vi "Parse Wiki.vi"(8 "error in":errorcluster, 9 "Parse from":enum16{"Proposal HTML:", "Proposal cluster"}(ring), 10 "Proposal Data":T2, 11 "Proposal document":path=path "C:/Users/l121767/Dropbox/Projects/FAIR/Project files/Proposal/National High Magnetic Field Laboratory - Users Program.html") -> (0 "error out":errorcluster, 3 "Puject  JSON":string)   [LabVIEW 2020]
uses:
  Utilities/iCalendar/Extract iCalendar String.ctl
  55103850-15ef-4a18-9388-7b0eadcdd449.vi
  <vilib>/JDP Science/JSONtext/Variant to JSON Text.vi
  <vilib>/JDP Science/JSONtext/LVClass Serializer/JSONtext LVClass Serializer.lvclass
panel:
  in  "OSF sub-project":T1={"data"={"type"="nodes", "attributes"={"title"="", "description"="", "public"=FALSE, "category"=""}}}
  in  "OSF Wiki":T3={"data"={"type"="wikis", "attributes"={"name"="", "content"=""}}}
  out "Proposal  title":string
  out "text":string
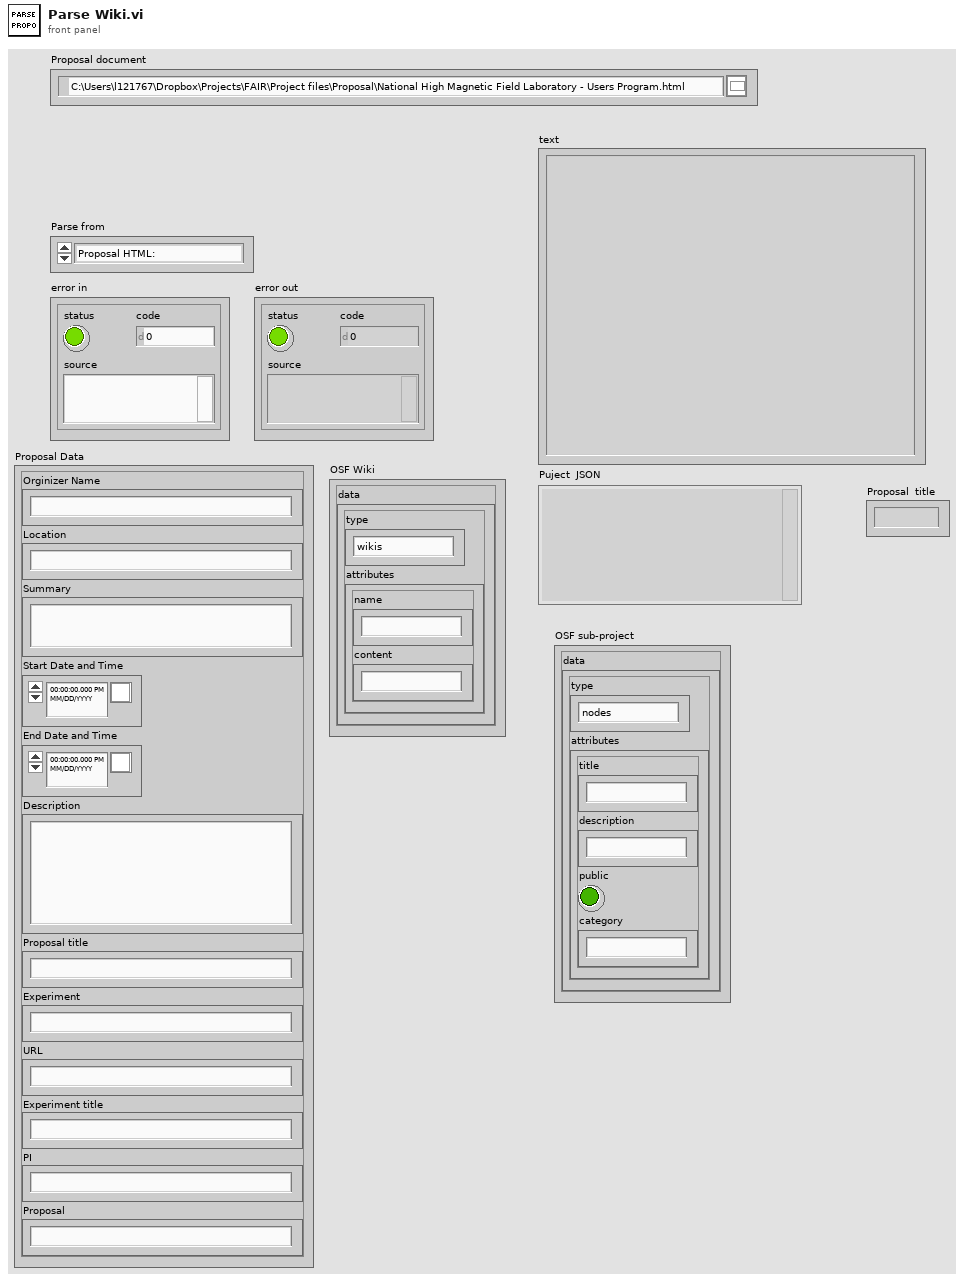
[diagram p1: front panel]
types:
  T1 = cluster{"data":cluster{"type":string, "attributes":cluster{"title":string, "description":string, "public":bool, "category":string}}}
  T2 = typedef "Extract iCalendar String.ctl" = cluster{"Orginizer Name":string, "Location":string, "Summary":string, "Start Date and Time":timestamp, "End Date and Time":timestamp, "Description":string, "Proposal title":string, "Experiment":string, "URL":string, "Experiment title":string, "PI":string, "Proposal":string}
  T3 = cluster{"data":cluster{"type":string, "attributes":cluster{"name":string, "content":string}}}
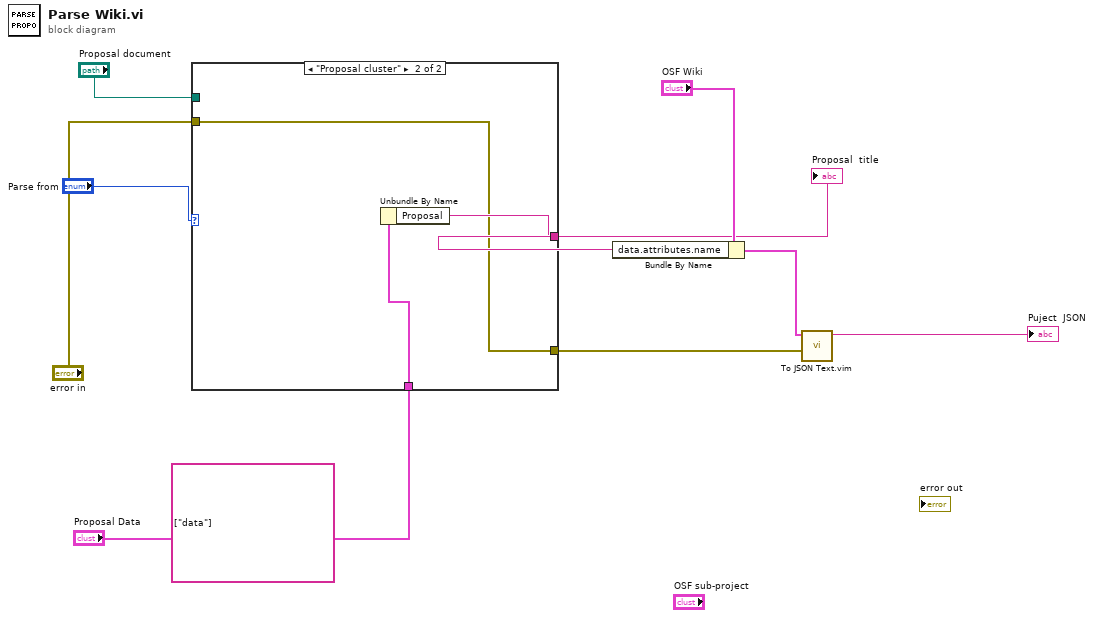
[diagram p0: block diagram]
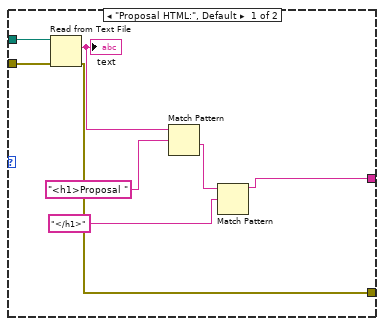
[diagram p2: hidden frame]
diagram:
  (unwired) string[] ["data"] ("Item Names")
  n1 = case shown="\"Proposal cluster\"" "Parse from" {
    tunnel: "Proposal document" -> [w17 _]
    tunnel: [w12 w19] -> w7
    tunnel: "error in" -> [w11 w18]
    tunnel: [w10 w18] -> w3
    tunnel: "Proposal Data" -> [_ w20]
    frame "Proposal HTML:", Default {
      n2 = Read from Text File(file (use dialog)=w17, error in=w11) -> (text=w16:string, error out=w10:errorcluster)  [unwired: 2 in, 2 out]
      "text" <- w16
      n3 = Match Pattern(string=w16, regular expression="<h1>Proposal ") -> (after substring=w14:string)  [unwired: 1 in, 3 out]
      n4 = Match Pattern(string=w14, regular expression="</h1>") -> (before substring=w12:string)  [unwired: 1 in, 3 out]
    }
    frame "Proposal cluster" {
      n5 = Unbundle By Name(w20) -> ("Proposal"=w19:string)
    }
  }
  "Proposal  title" <- w7
  n6 = Bundle By Name(cluster="OSF Wiki", "data.attributes.name"=w7) -> (w6:T3)
  n7 = call "To JSON Text.vim"("error in (no error)"=w3, "Anything"=w6) -> ("<JSON>"=→"Puject  JSON":string)  [unwired: 8 in, 1 out]
